vi "GESTORE PROFILI.vi"() -> ()   [LabVIEW 2019]
uses:
  GESTIONE PROFILI Folder/controls/STEP.ctl
  GESTIONE PROFILI Folder/controls/Caratteristiche step.ctl
  TypeDef/PROCEDURE.ctl
  Stato comandi freno.vi
  Stato alimentatore 1.vi
  Global stato profilo.vi
  Acq avvenuta global.vi
  Global CAMBIO CTRL FRENO.vi
  Global Gestione stop se eq termico.vi
  Global procedura abilitata.vi
  Global Fine procedure.vi
  <vilib>/addons/database/NI_Database_API.lvlib
panel:
  in  "To Select Wait":bool=TRUE
  in  "milliseconds to wait":u32=5000
  out "appended array":timestamp[](array[timestamp])
  out "UTILIZZO BANCO":T1(ring)
  out "Settings profilo":T2
  out "Cluster 2":T3
  in  "AGGIORNA SETTINGS AVVIO":bool
  in  "Modalità avvio":T4={"MODALITA' BANCO"=enum."SOLO FRENO", "MODALITA' AVVIO MOTORE"=enum."AVVIO DIRETTO DA LINEA", "MODALITA' AVVIO FRENO"=enum."MARCIA DOPO AVVIO MOTORE", "V avvio[V]"=0.0, "F avvio[Hz]"=0.0, "%V ridotta"=0.0, "C avvio [Nm]"=0.0, "RPM avvio"=0.0, "SERVO AVVIO"=FALSE, "SENSO DI ROTAZIONE"=FALSE}
  in  "NOME PROFILO":string
  in  "CARICA PROFILO":bool
  out "data":T5
  in  "AGGIORNA DATI NOMINALI":bool
  in  "Data":T5
  out "State Called in Queue":string
  in  "EXIT":bool
  in  "Stop Button":bool
  in  "Pause Button":bool
  in  "Play Button":bool
  in  "StatoEsegui":string
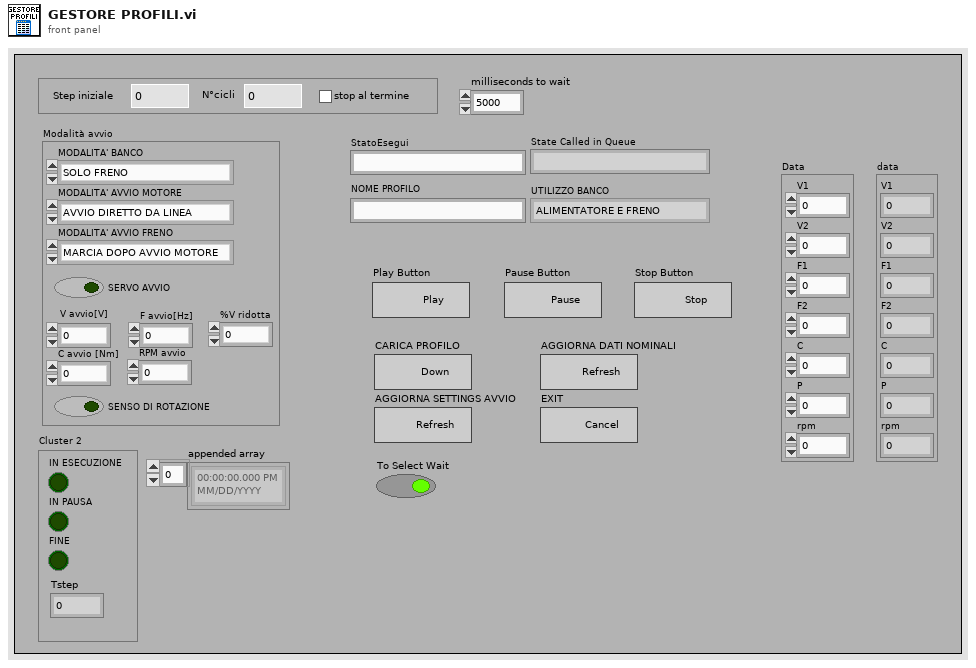
[diagram p1: front panel]
types:
  T1 = enum32{"ALIMENTATORE E FRENO", "SOLO ALIMENTATORE", "SOLO FRENO (TRASCINAMENTO)", "GESTIONE MANUALE", "SOLO ACQUISITORE", "VARIAC"}
  T2 = cluster{"Step iniziale":dbl, "N°cicli":dbl, "stop al termine":bool}
  T3 = cluster{"IN ESECUZIONE":bool, "IN PAUSA":bool, "FINE":bool, "Tstep":dbl}
  T4 = typedef "Modalità avvio.ctl" = cluster{"MODALITA' BANCO":enum32{"ALIMENTATORE E FRENO", "SOLO ALIMENTATORE", "SOLO FRENO", "GESTIONE MANUALE", "SOLO ACQUISITORE", "VARIAC"}, "MODALITA' AVVIO MOTORE":enum32{"AVVIO A TENSIONE RIDOTTA", "AVVIO IN RAMPA", "AVVIO DIRETTO DA ALIM", "AVVIO DIRETTO DA LINEA"}, "MODALITA' AVVIO FRENO":enum32{"MARCIA DOPO AVVIO MOTORE", "MARCIA PRIMA AVVIO"}, "V avvio[V]":dbl, "F avvio[Hz]":dbl, "%V ridotta":dbl, "C avvio [Nm]":dbl, "RPM avvio":dbl, "SERVO AVVIO":bool, "SENSO DI ROTAZIONE":bool}
  T5 = cluster{"V1":dbl, "V2":dbl, "F1":dbl, "F2":dbl, "C":dbl, "P":dbl, "rpm":dbl}
  T6 = cluster{"Message":string, "Message Data":variant}
  T7 = typedef "STEP.ctl" = cluster{"Tipo prova":string, "Misura resistenza ?":bool, "Tempo Step[s]":dbl, "Freno":cluster{"MARCIA":bool, "Control Type":enum32{"Torque [Nm]", "Power [W]", "Speed [RPM]", "Corrente [A]"}, "RIF %":dbl}, "ALIMENTATORE 1":cluster{"MARCIA":bool, "RIF V":dbl, "RIF F":dbl}, "ALIMENTATORE 2":cluster{"MARCIA":bool, "RIF V":dbl, "RIF F":dbl}, "Caratteristiche step":T8}
  T8 = typedef "Caratteristiche step.ctl" = cluster{"Attendi stabilizz.":bool, "Acq. fine step?":bool, "Acq. automatiche":bool, "PID FRENO":bool, "PID ALIMENTATORE 1":bool, "PID ALIMENTATORE 2":bool, "CAMBIA PROVA SE EQ. TERMICO":bool}
  T9 = cluster{"#ripetizione in corso":i32, "Step in corso":i32}
  T10 = cluster{"Array of elements":cluster{"String":string, "variant":variant}[], "Single element":cluster{"String":string, "variant":variant}, "enque at\nopposite end (F)":bool, "no replications (F)":bool}
  T11 = cluster{"N°Acq":i16, "Periodo":dbl, "acq in corso":bool, "Acquisizione":bool, "Slide":u8, "Inserisci Acq.":bool, "Elimina riga":bool, "Acq auto":bool, "Intervallo":dbl}
  T12 = typedef "PROCEDURE.ctl" = enum16{"START", "STOP AUTOMATICO", "STOP FRENO", "ABILITA POTENZA", "DISABILITA POTENZA", "CHIUDI POTENZA", "APRI POTENZA", "MISURA RESISTENZA RESISTOMAT", "PROVA ROTORE BLOCCATO", "MISURA RESISTENZA RES METER", "START AFE ALTERNATORI", "STOP AFE ALTERNATORI", "STOP ALIMENTATORE", "CONFIG CONTROLLO FRENO", "ALLARME", "START PROFILO", "SVUOTA BUFFER PROCEDURE E OPERAZIONI"}
  T13 = cluster{"Step iniziale":i32, "N°cicli":i32, "stop al termine":bool}
  T14 = typedef "Stato inverter selezionato.ctl" = cluster{"Stato comandi freno":T15, "Stato":cluster{"rif C%":dbl, "rif vel%":dbl, "Controllo effettivo":enum32{"Torque [Nm]", "Power [W]", "Speed [RPM]"}, "Controllo desiderato":enum32{"Torque [Nm]", "Power [W]", "Speed [RPM]"}, "Fine rampa C":bool, "Fine rampa RPM":bool, "Senso rotaz":bool, "Start":bool, "C stabile":bool, "P stabile":bool, "RPM stabile":bool}}
  T15 = typedef "Comandi freno.ctl" = cluster{"Control":cluster{"Control Type":enum32{"Torque [Nm]", "Power [W]", "Speed [RPM]", "Corrente [A]"}, "Set":dbl, "Inverti senso di rotazione":bool}, "Start\\stop":cluster{"Start":bool, "STOP":bool}, "Status":cluster{"Ready":bool, "Running":bool, "Regulation":bool}, "PID":bool, "Abilita":cluster{"Abilita":bool}, "Status ref":cluster{"Torque":dbl, "Speed":dbl}}
  T16 = typedef "Comandi_Alimentatore.ctl" = cluster{"RIF 1":dbl, "RIF 2":dbl, "Status":cluster{"Ready":bool, "Running":bool, "Regulation":bool}, "Start\\stop":cluster{"Start":bool, "Stop":bool}, "PID RIF1":bool, "PID RIF2":bool, "Status ref":cluster{"RIF 1":dbl, "RIF 2":dbl}, "Abilita":cluster{"Abilita":bool}}
  T17 = cluster{"RIF 1":dbl, "RIF 2":dbl, "Abilitato":bool, "In marcia":bool, "Fine rampa RIF1":bool, "Fine rampa RIF2":bool, "Vstabile":bool, "F stabile":bool, "PID RIF1":bool, "PID RIF2":bool, "Alimentatore 1":T16}
  T18 = cluster{"RIF 1":dbl, "RIF 2":dbl, "Abilitato":bool, "In marcia":bool, "Fine rampa RIF1":bool, "Fine rampa RIF2":bool, "Vstabile":bool, "F stabile":bool, "PID RIF1":bool, "PID RIF2":bool, "Alimentatore 2":T16}
  T19 = typedef "NI_Database_API.lvlib/Conn ObjectReference.ctl" = refnum<k1>
  T20 = enum32{"Torque [Nm]", "Power [W]", "Speed [RPM]", "Corrente [A]"}
  T21 = cluster{"Caratteristiche step":T8, "Step profilo":string[][]}
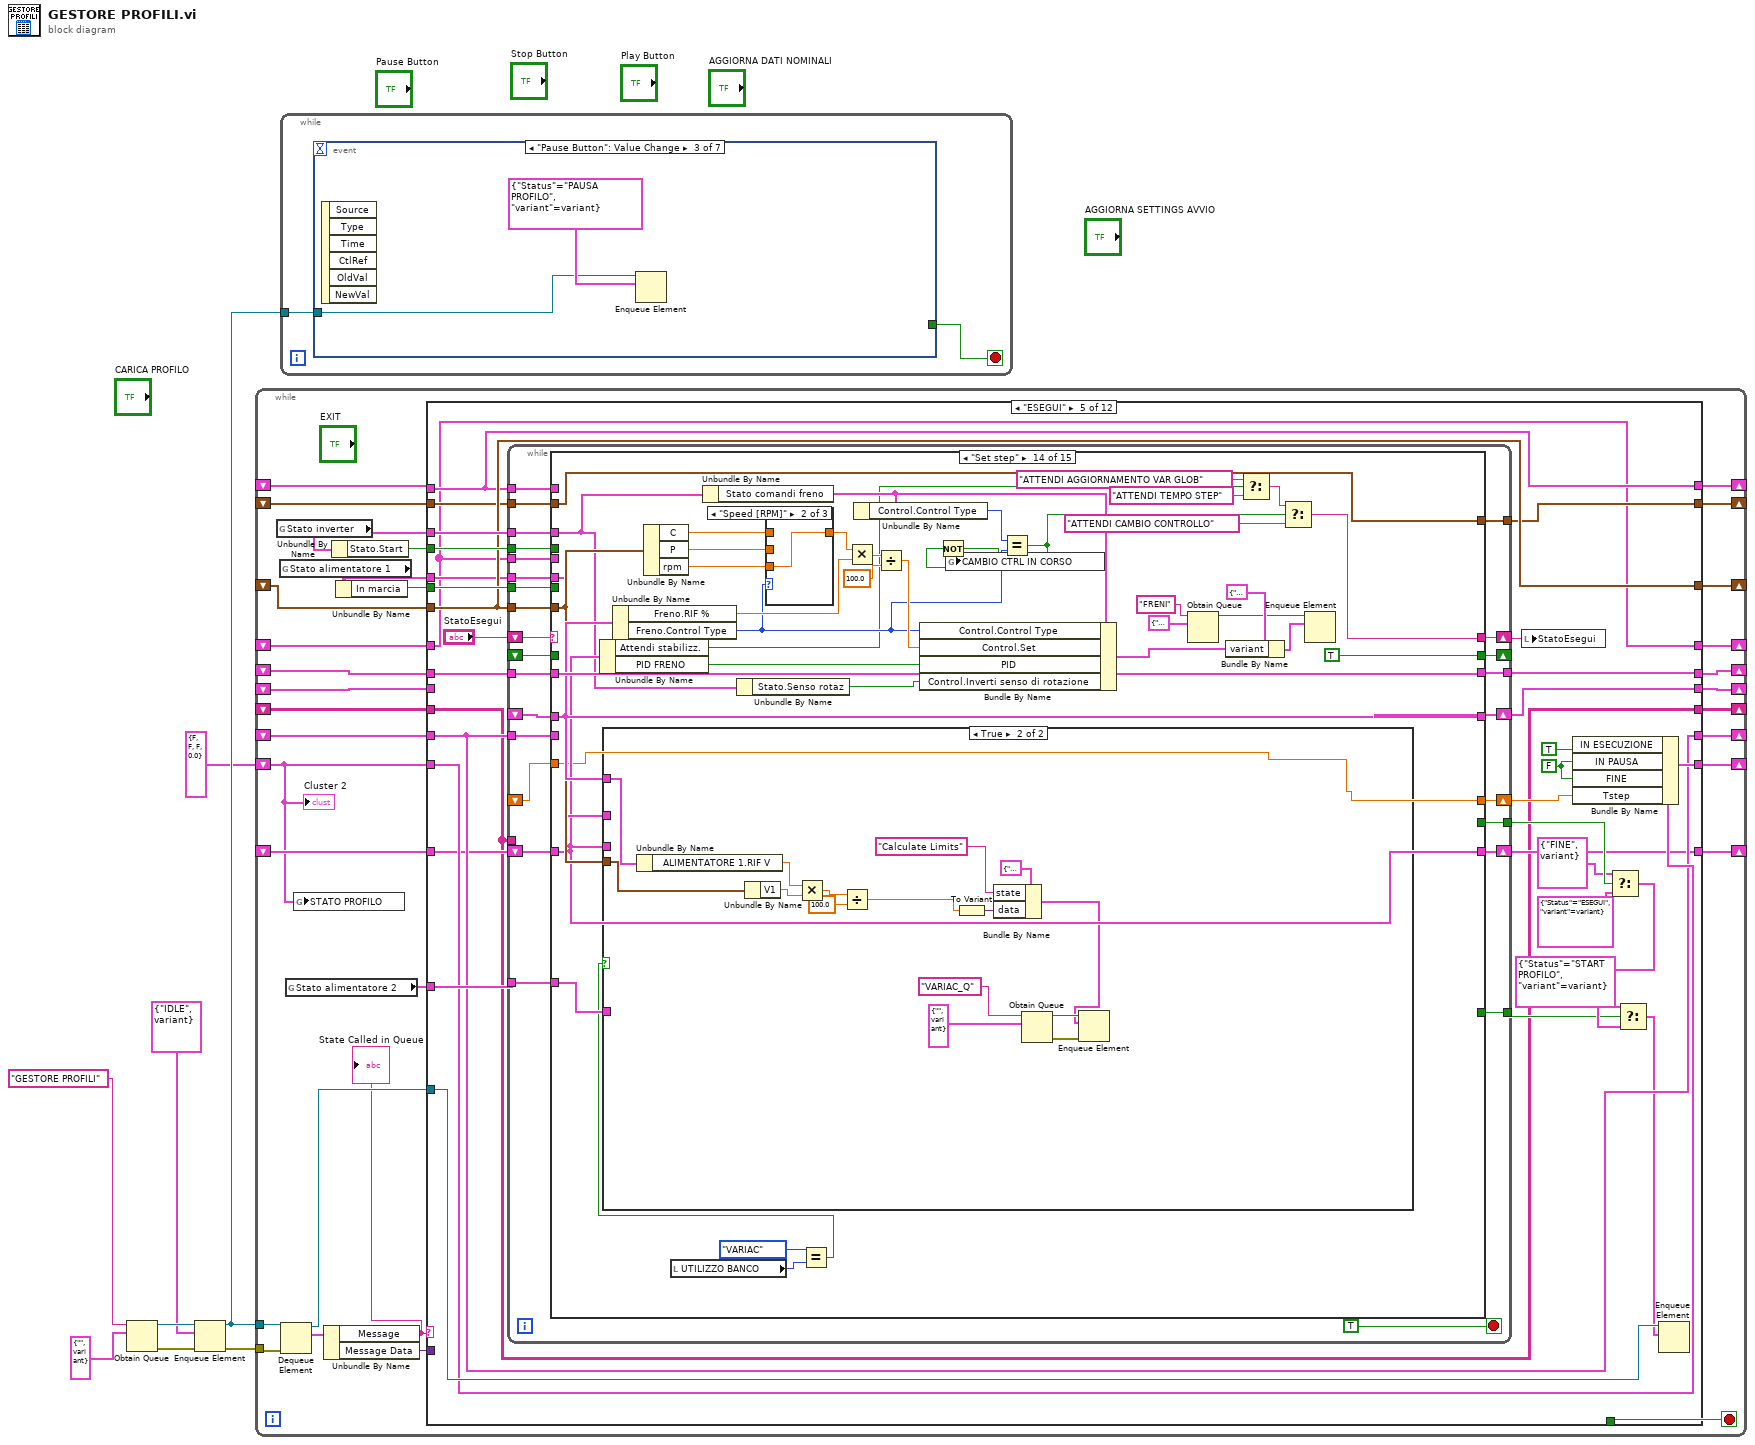
[diagram p0: block diagram]
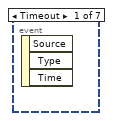
[diagram p2: hidden frame]
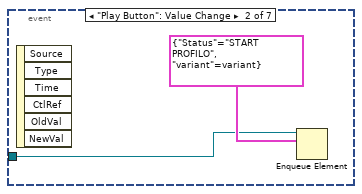
[diagram p3: hidden frame]
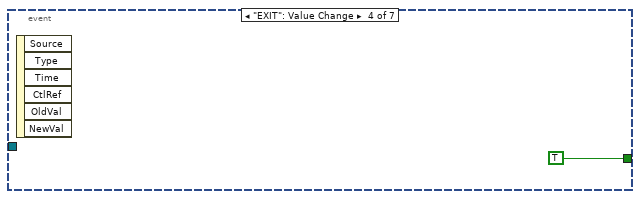
[diagram p4: hidden frame]
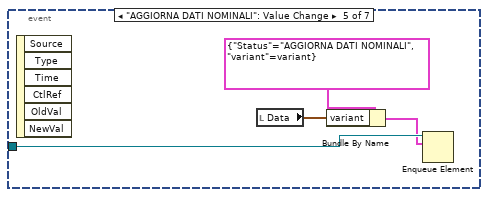
[diagram p5: hidden frame]
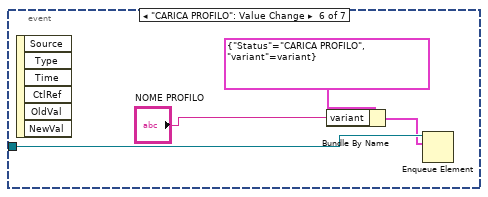
[diagram p6: hidden frame]
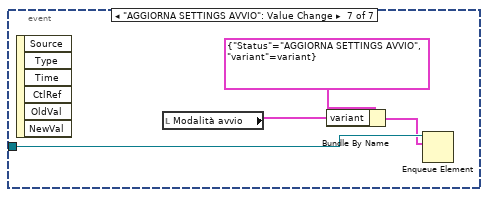
[diagram p7: hidden frame]
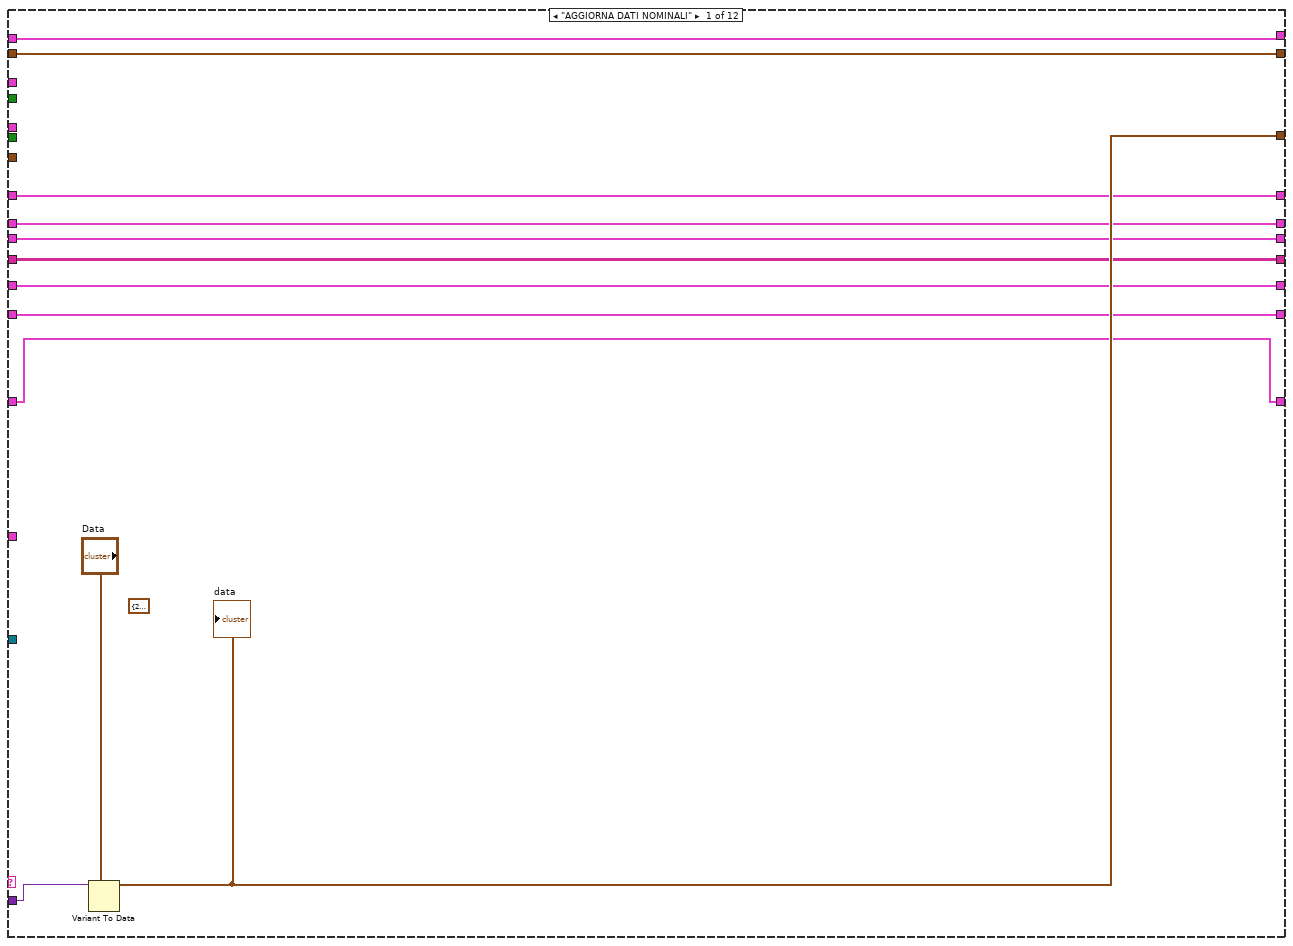
[diagram p8: hidden frame]
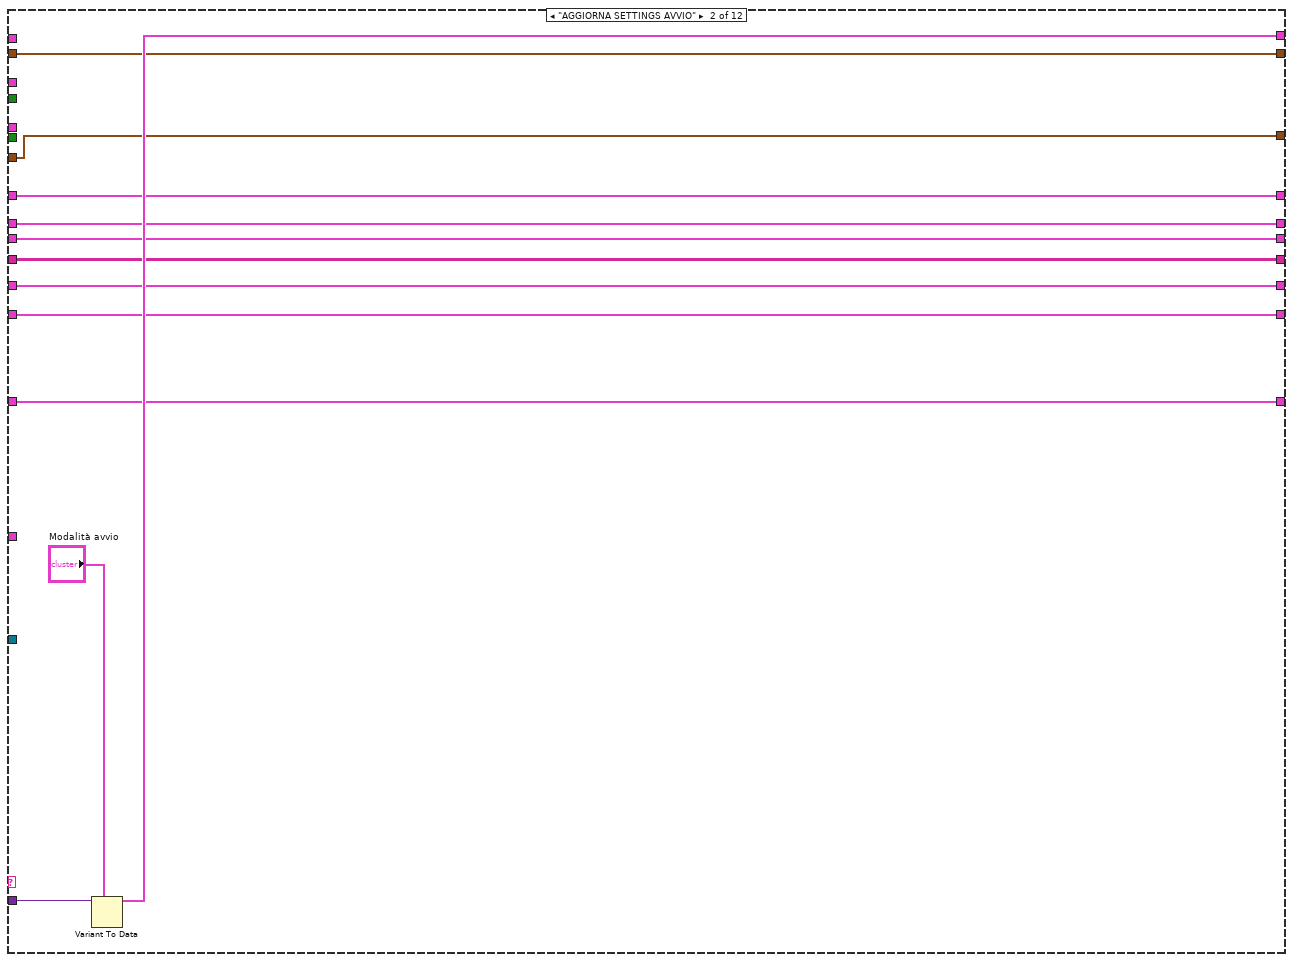
[diagram p9: hidden frame]
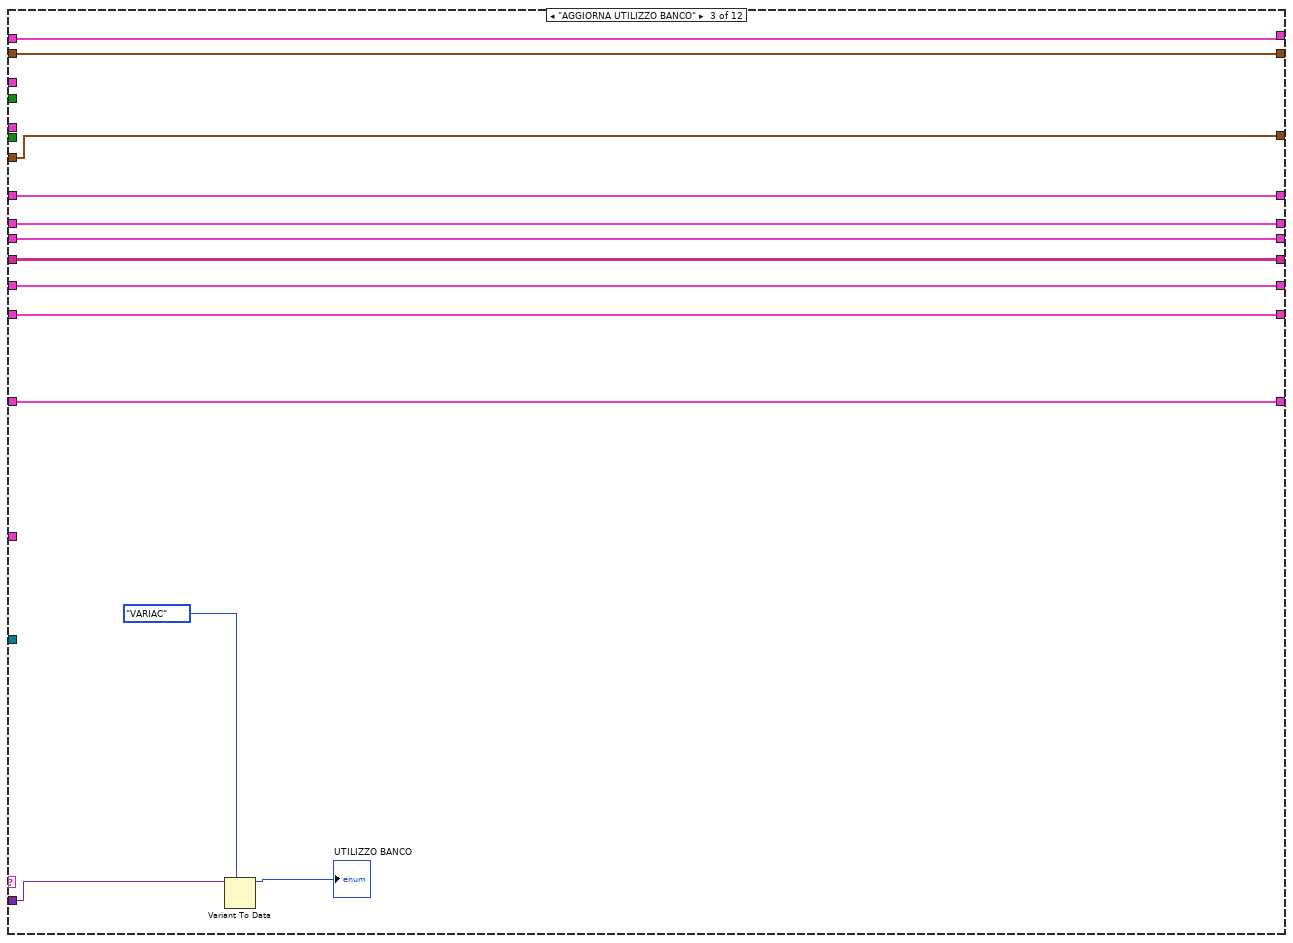
[diagram p10: hidden frame]
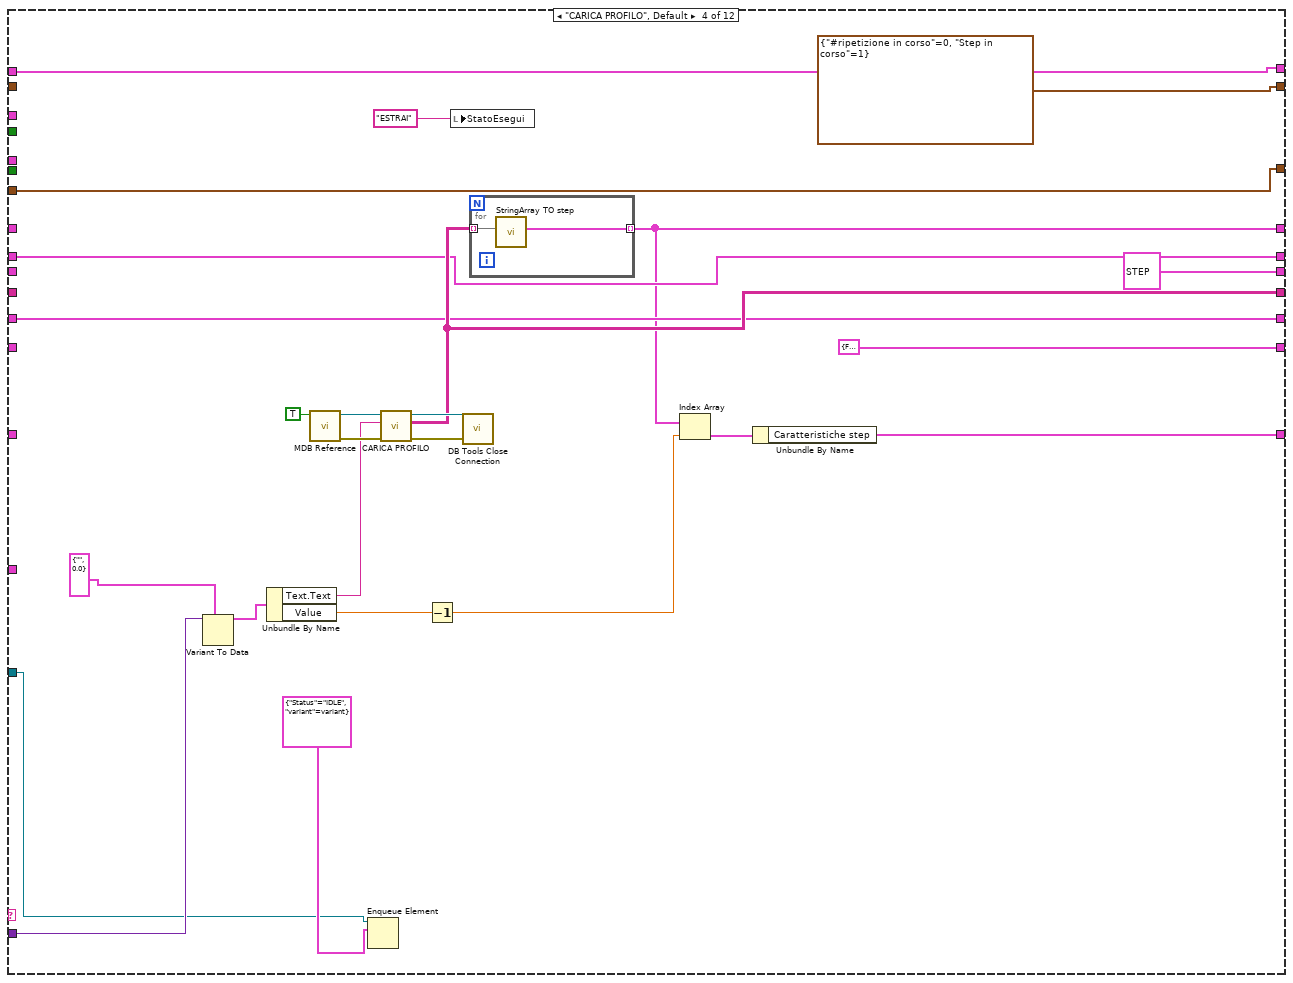
[diagram p11: hidden frame]
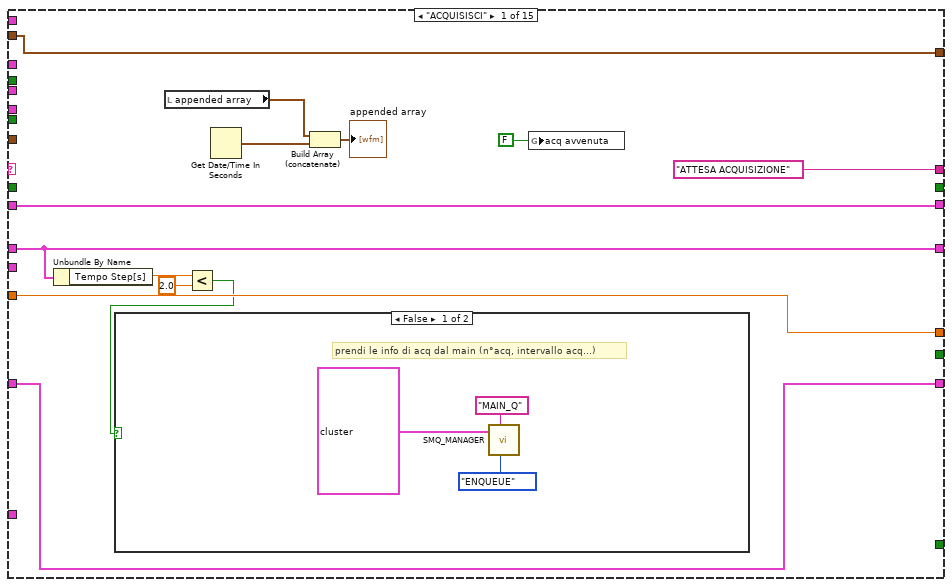
[diagram p12: hidden frame]
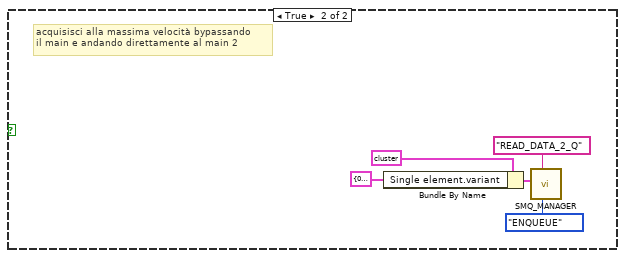
[diagram p13: hidden frame]
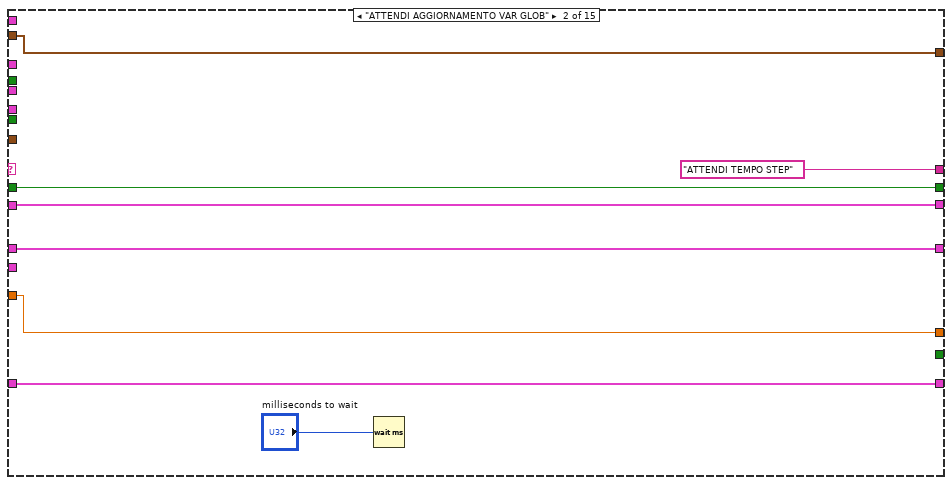
[diagram p14: hidden frame]
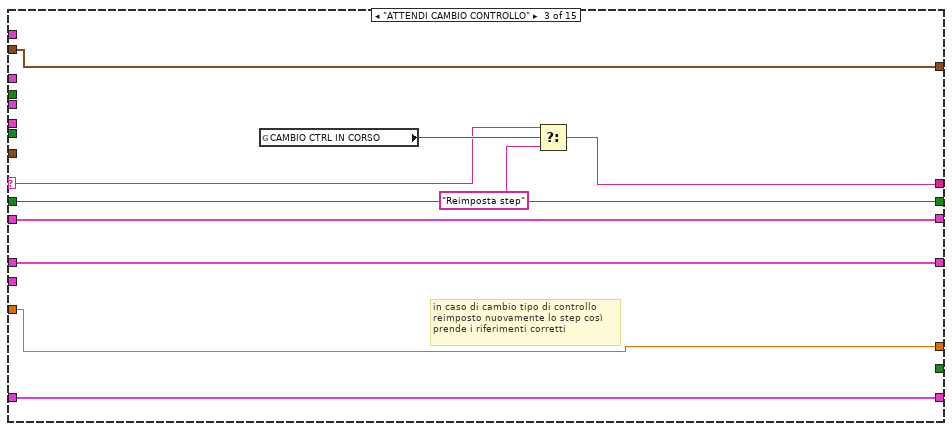
[diagram p15: hidden frame]
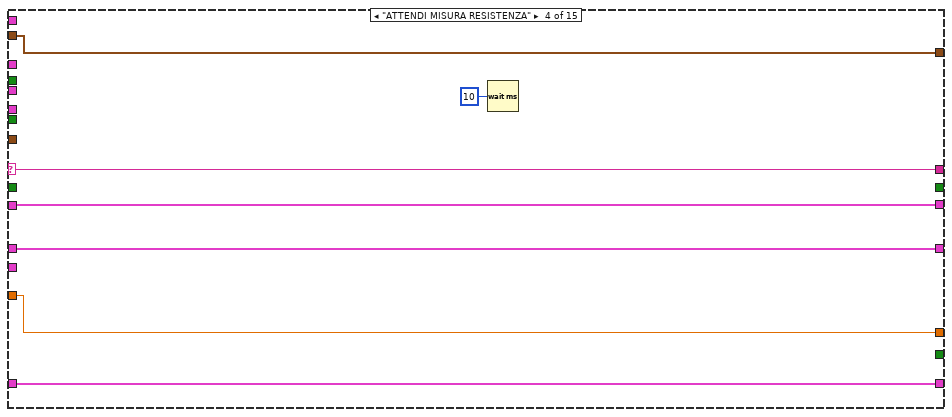
[diagram p16: hidden frame]
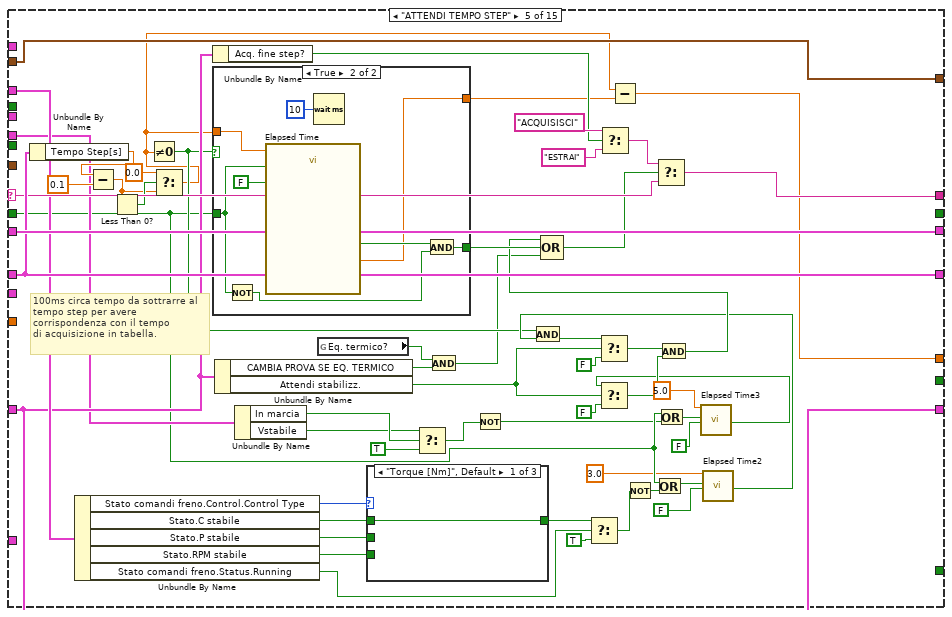
[diagram p17: hidden frame]
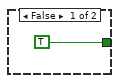
[diagram p20: hidden frame]
diagram:
  n1 = Obtain Queue(name (unnamed)="GESTORE PROFILI", element data type=T6 {"Message"="", "Message Data"=variant} ("Message Cluster")) -> (queue out=w7:refnum<queue>, error out=w8:errorcluster)  [unwired: 3 in, 1 out]
  n2 = Enqueue Element(queue=w7, element=cluster{"Status":string, "variant":variant} {"Status"="IDLE", "variant"=variant}, error in (no error)=w8) -> (queue out=w2:refnum<queue>, error out=w3:errorcluster)  [unwired: 1 in, 1 out]
  n3 = while {
    shift-right: [w40] -> _
    shift-left: _ -> [w39]
    shift-right: [w34] -> _
    shift-left: _ -> [w33]
    tunnel: w2 -> [w32]
    tunnel: w3 -> [w31]
    shift-right: [w25] -> _
    shift-left: _ -> [w24]
    shift-right: [w23] -> _
    shift-left: _ -> [w22]
    shift-right: [w20] -> _
    shift-left: _ -> [w19]
    shift-right: [w18] -> _
    shift-left: _ -> [w17]
    shift-right: [w16] -> _
    shift-left: T3 {"IN ESECUZIONE"=FALSE, "IN PAUSA"=FALSE, "FINE"=FALSE, "Tstep"=0.0} ("STATO PROFILO") -> [w11]
    shift-right: [w15] -> _
    shift-left: _ -> [w14]
    shift-right: [w13] -> _
    shift-left: _ -> [w12]
    shift-right: [w10] -> _
    shift-left: _ -> [w9]
    stop <- w27 stop-if-true
    n4 = global read "Stato comandi freno.vi" "Stato inverter"() -> (w36:T14)
    n5 = global read "Stato alimentatore 1.vi" "Stato alimentatore 1"() -> (w35:T17)
    n6 = Dequeue Element(queue=w32, error in (no error)=w31) -> (queue out=w28:refnum<queue>, element=w30:T6)  [unwired: 1 in, 2 out]
    n7 = global read "Stato alimentatore 1.vi" "Stato alimentatore 2"() -> (w26:T18)
    n8 = global write "Global stato profilo.vi" "STATO PROFILO"(w11) -> ()
    n9 = Unbundle By Name(w30) -> ("Message"=w21:string, "Message Data"=w29:variant)
    "State Called in Queue" <- w21
    n10 = Unbundle By Name(w36) -> ("Stato.Start"=w38:bool)
    n11 = Unbundle By Name(w35) -> ("In marcia"=w37:bool)
    n12 = case shown="\"ESEGUI\"" w21 {
      tunnel: [w45 w61 w69 w90 w135 w594 w611 w625 w646 w651 w672 T7[] []] -> w40
      tunnel: w39 -> [w45 w61 w69 w90 w136 w594 w611 w625 w646 w651 w673 _]
      tunnel: w38 -> [_ _ _ _ w134 _ _ _ _ _ _ _]
      tunnel: w37 -> [_ _ _ _ w133 _ _ _ _ _ _ _]
      tunnel: w36 -> [_ _ _ _ w132 _ _ _ _ _ _ _]
      tunnel: w24 -> [_ w60 w77 w100 w131 w593 w609 w632 w644 w659 w678 w706]
      tunnel: w35 -> [_ _ _ _ w130 _ _ _ _ _ _ _]
      tunnel: w33 -> [w49 _ w70 w102 w129 w595 w612 w633 w647 w653 w671 w699]
      tunnel: [w49 w62 w70 w102 w129 w595 w612 w633 w647 w653 w671 w699] -> w34
      tunnel: w29 -> [w52 w64 w71 w94 _ _ _ _ _ w655 _ _]
      tunnel: w28 -> [_ _ _ w92 w127 _ w610 _ w645 _ w679 w695]
      tunnel: [_ _ _ _ _ w591 _ _ _ _ _ _] -> w27
      tunnel: w26 -> [_ _ _ _ w122 _ _ _ _ _ _ _]
      tunnel: [w50 w60 w77 w100 w131 w593 w609 w632 w644 w659 w678 w706] -> w25
      tunnel: [w48 w59 w76 w85 w106 w592 w599 w626 w643 w658 w670 w705] -> w23
      tunnel: w22 -> [w48 w59 w76 _ w107 w592 w599 w626 w643 w658 w670 w705]
      tunnel: [w47 w58 w75 w91 w105 w590 w608 w624 w642 w657 w677 w704] -> w20
      tunnel: w19 -> [w47 w58 w75 _ w105 w590 w608 w624 w642 w657 w677 w704]
      tunnel: [w46 w57 w74 w87 w114 w589 w605 w623 w641 w656 w665 w703] -> w18
      tunnel: w17 -> [w46 w57 w74 _ w114 w589 w605 w623 w641 w656 w665 w703]
      tunnel: w11 -> [w44 w56 w68 _ w121 w588 w604 w622 w640 w650 w675 w702]
      tunnel: [w44 w56 w68 T3 {"IN ESECUZIONE"=FALSE, "IN PAUSA"=FALSE, "FINE"=FALSE, "Tstep"=0.0} ("STATO PROFILO") w120 w588 w603 w622 w639 w650 w675 w702] -> w16
      tunnel: [w43 w54 w73 w88 w117 w586 w598 w620 w635 w652 w663 w698] -> w15
      tunnel: w14 -> [w43 w54 w73 w88 w117 w586 w598 w620 w635 _ w663 w698]
      tunnel: [w41 w55 w72 T9 {"#ripetizione in corso"=0, "Step in corso"=1} w115 w587 w600 w621 w636 w649 w662 T9 {"#ripetizione in corso"=0, "Step in corso"=1}] -> w13
      tunnel: w12 -> [w41 w55 w72 _ w116 w587 w600 w621 w636 w649 w662 _]
      tunnel: [w42 w53 w67 T7 {"Tipo prova"="[3] ROT. BLOCCATO", "Misura resistenza ?"=FALSE, "Tempo Step[s]"=0.0, "Freno"={"MARCIA"=FALSE, "Control Type"=enum."Torque [Nm]", "RIF %"=0.0}, "ALIMENTATORE 1"={"MARCIA"=FALSE, "RIF V"=0.0, "RIF F"=0.0}, "ALIMENTATORE 2"={"MARCIA"=FALSE, "RIF V"=0.0, "RIF F"=0.0}, "Caratteristiche step"={"Attendi stabilizz."=TRUE, "Acq. fine step?"=TRUE, "Acq. automatiche"=TRUE, "PID FRENO"=TRUE, "PID ALIMENTATORE 1"=TRUE, "PID ALIMENTATORE 2"=FALSE, "CAMBIA PROVA SE EQ. TERMICO"=FALSE}} ("STEP") w108 w585 w596 w619 w634 w648 w666 w694] -> w10
      tunnel: w9 -> [w42 w53 w67 _ _ w585 w596 w619 w634 w648 w666 w694]
      frame "AGGIORNA DATI NOMINALI" {
        (unwired) T5 {"V1"=250.0, "V2"=0.0, "F1"=50.0, "F2"=0.0, "C"=25.0, "P"=10.0, "rpm"=2100.0} ("Cluster")
        n13 = Variant To Data(type="Data", Variant=w52) -> (data=w50:T5)  [unwired: 1 in, 1 out]
        "data" <- w50
      }
      frame "AGGIORNA SETTINGS AVVIO" {
        n14 = Variant To Data(type="Modalità avvio", Variant=w64) -> (data=w62:T4)  [unwired: 1 in, 1 out]
      }
      frame "AGGIORNA UTILIZZO BANCO" {
        n15 = Variant To Data(type=T1."VARIAC" ("MODALITA' UTILIZZO BANCO"), Variant=w71) -> (data=→"UTILIZZO BANCO":T1)  [unwired: 1 in, 1 out]
      }
      frame "CARICA PROFILO", Default {
        n16 = Variant To Data(type=cluster{"Text.Text":string, "Value":dbl} {"Text.Text"="", "Value"=0.0} ("output cluster"), Variant=w94) -> (data=w81:cluster{"Text.Text":string, "Value":dbl})  [unwired: 1 in, 1 out]
        n17 = Unbundle By Name(w81) -> ("Text.Text"=w80:string, "Value"=w79:dbl)
        n18 = call "MDB Reference.vi"("Collaudi T/motori F"=TRUE) -> ("error out"=w98:errorcluster, "Refnum out"=w96:T19)  [unwired: 8 in, 1 out]
        n19 = Enqueue Element(queue=w92, element=cluster{"Status":string, "variant":variant} {"Status"="IDLE", "variant"=variant}) -> ()  [unwired: 2 in, 3 out]
        n20 = call "CARICA PROFILO.vi"("error in (no error)"=w98, "Text.Text"=w80, "Refnum in"=w96) -> ("error out"=w97:errorcluster, "Step profilo"=w91:string[][], "Refnum out"=w95:T19)  [unwired: 3 in, 3 out]
        n21 = Decrement(x=w79) -> (x-1=w78:dbl)
        n22 = local write "StatoEsegui"("ESTRAI" ("StatoEsegui")) -> ()
        n23 = call <vilib>:"DB Tools Close Connection.vi"("error in (no error)"=w97, "connection reference"=w95) -> ()  [unwired: 5 in, 1 out]
        n24 = for {
          tunnel: w91 -> [w104] mode=indexing
          tunnel: [w103] -> w87 mode=indexing
          n25 = call "StringArray TO step.vi"("ItemNames"=w104) -> ("STEP"=w103:T7)  [unwired: 10 in]
        }
        n26 = Index Array(array=w87, index=w78) -> (element=w86:T7)
        n27 = Unbundle By Name(w86) -> ("Caratteristiche step"=w85:T8)
      }
      frame "ESEGUI" {
        w118 = FALSE ("IN PAUSA")
        n28 = while {
          shift-right: [w154] -> w123
          shift-left: "StatoEsegui" -> [w162]
          tunnel: w136 -> [w160]
          tunnel: [w159] -> w135
          shift-right: [w158] -> w108
          shift-left: _ -> [w157]
          tunnel: w134 -> [w156]
          tunnel: w133 -> [w155]
          tunnel: w132 -> [w153]
          tunnel: w131 -> [w152]
          tunnel: w130 -> [w151]
          tunnel: w129 -> [w150]
          tunnel: [w149] -> w128
          shift-right: [w148] -> _
          shift-left: _ -> [w147]
          tunnel: w122 -> [w146]
          tunnel: w117 -> [w144]
          tunnel: w116 -> [w143]
          tunnel: [w142] -> w115
          tunnel: w114 -> [w141]
          tunnel: [w140] -> w111
          shift-right: [w138] -> w106
          shift-left: w107 -> [w145]
          shift-right: [w139] -> w109
          shift-left: _ -> [w137]
          tunnel: w105 -> [_]
          stop <- TRUE stop-if-true
          n29 = case shown="\"Set step\"" w162 {
            selector: w162 -> [_ _ w196 w203 w261 w284 _ w359 w365 _ _ w407 _ _ w583]
            tunnel: w160 -> [w175 w186 w199 w205 w264 w285 w323 w358 w364 w381 w399 w406 w472 w515 w580]
            tunnel: [w175 w186 w199 w205 w264 w285 w331 w358 w364 w381 w399 w406 w472 w515 w580] -> w159
            tunnel: [w166 w185 w200 w206 w263 w286 w290 w357 w363 w375 w398 w405 w439 w505 w579] -> w158
            tunnel: w157 -> [w166 w185 w200 w206 w263 w286 _ w357 w363 w375 w398 w405 w439 w505 w579]
            tunnel: w156 -> [_ _ _ _ _ _ _ _ _ _ _ _ _ _ _]
            tunnel: w155 -> [_ _ _ _ _ _ _ _ _ _ _ _ _ _ _]
            tunnel: ["ATTESA ACQUISIZIONE" ("t") "ATTENDI TEMPO STEP" ("t") w195 w203 w260 w283 w294 w359 w365 w372 "ATTENDI MISURA RESISTENZA" ("t") w407 "ATTENDI AGGIORNAMENTO VAR GLOB" ("t") w489 w582] -> w154
            tunnel: w153 -> [_ _ _ _ w255 _ _ _ _ w379 _ _ w471 w485 _]
            tunnel: w152 -> [_ _ _ _ _ _ _ _ _ w377 _ _ w438 w504 _]
            tunnel: w151 -> [_ _ _ _ w217 _ _ _ _ w378 _ _ w437 w503 _]
            tunnel: w150 -> [_ _ _ _ _ _ _ _ _ w380 _ _ _ _ _]
            tunnel: [_ _ _ _ _ _ _ TRUE _ _ _ _ _ _ _] -> w149
            tunnel: [_ w187 w198 _ _ _ _ _ _ _ _ _ TRUE TRUE _] -> w148
            tunnel: w147 -> [_ w187 w198 _ w216 _ _ _ _ _ _ _ _ _ _]
            tunnel: w146 -> [_ _ _ _ _ _ _ _ _ _ _ _ w436 w502 _]
            tunnel: w145 -> [w171 w189 w193 w207 w253 w278 w311 w354 w361 _ w400 w403 w415 w494 w576]
            tunnel: w144 -> [_ _ _ _ _ _ w336 _ _ _ _ _ _ _ _]
            tunnel: w143 -> [w172 w191 w201 w208 w254 w279 w328 w355 w362 w376 w401 w408 w413 w493 w577]
            tunnel: [w172 w191 w201 w208 w254 w279 w333 w355 w362 w376 w401 w408 w413 w493 w577] -> w142
            tunnel: w141 -> [_ _ _ _ _ _ w332 _ _ _ _ _ _ _ _]
            tunnel: [_ _ _ _ _ _ _ _ _ _ _ TRUE _ _ _] -> w140
            tunnel: [w170 w190 w192 w202 w228 w277 0.0 w353 w360 w371 w393 w402 w409 w483 w575] -> w139
            tunnel: [w171 w189 w193 w207 w253 w278 w311 w354 w361 w374 w400 w403 w415 w494 w576] -> w138
            tunnel: w137 -> [w170 w190 w192 w202 _ w277 _ w353 w360 w371 w393 w402 w409 w483 w575]
            frame "ACQUISISCI" {
              n30 = Unbundle By Name(w166) -> ("Tempo Step[s]"=w165:dbl)
              n31 = local read "appended array"() -> (w167:timestamp[])
              n32 = Less?(x=w165, y=2.0) -> (x < y?=w163:bool)
              n33 = case shown="False" w163 {
                frame False {
                  # "prendi le info di acq dal main (n°acq, intervallo acq...)"
                  n34 = call <userlib>:"SMQ_MANAGER.vi"("Function"=enum16{"INITIALIZE", "ENQUEUE", "STOP ALL"}."ENQUEUE", "Queue name"="MAIN_Q", "Enqueue cluster"=T10 {"Array of elements"=[], "Single element"={"String"="ACQUISISCI", "variant"=variant}, "enque at\nopposite end (F)"=FALSE, "no replications (F)"=FALSE}) -> ()  [unwired: 8 in, 1 out]
                }
                frame True {
                  # "acquisisci alla massima velocità bypassando\nil main e andando direttamente al main 2"
                  n35 = Bundle By Name(cluster=T10 {"Array of elements"=[], "Single element"={"String"="START ACQ", "variant"=variant}, "enque at\nopposite end (F)"=FALSE, "no replications (F)"=FALSE} ("Enqueue cluster"), "Single element.variant"=T11 {"N°Acq"=0, "Periodo"=0.0, "acq in corso"=FALSE, "Acquisizione"=FALSE, "Slide"=2, "Inserisci Acq."=FALSE, "Elimina riga"=FALSE, "Acq auto"=FALSE, "Intervallo"=5.0} ("Acquisizioni")) -> (w180:T10)
                  n36 = call <userlib>:"SMQ_MANAGER.vi"("Function"=enum16{"INITIALIZE", "ENQUEUE", "STOP ALL"}."ENQUEUE", "Queue name"="READ_DATA_2_Q", "Enqueue cluster"=w180) -> ()  [unwired: 8 in, 1 out]
                }
              }
              n37 = Get Date/Time In Seconds() -> (seconds since 1Jan1904=w169:timestamp)
              n38 = Build Array (concatenate)(w167, w169) -> (→"appended array":timestamp[])
              n39 = global write "Acq avvenuta global.vi" "acq avvenuta"(FALSE) -> ()
            }
            frame "ATTENDI AGGIORNAMENTO VAR GLOB" {
              n40 = Wait (ms)(milliseconds to wait="milliseconds to wait") -> ()  [unwired: 1 out]
            }
            frame "ATTENDI CAMBIO CONTROLLO" {
              # "in caso di cambio tipo di controllo\nreimposto nuovamente lo step così\nprende i riferimenti corretti"
              n41 = global read "Global CAMBIO CTRL FRENO.vi" "CAMBIO CTRL IN CORSO"() -> (w197:bool)
              n42 = Select(t=w196, s=w197, f="Reimposta step") -> (s? t:f=w195:string)
            }
            frame "ATTENDI MISURA RESISTENZA" {
              n43 = Wait (ms)(milliseconds to wait=u32 10) -> ()  [unwired: 1 out]
            }
            frame "ATTENDI TEMPO STEP" {
              # "100ms circa tempo da sottrarre al\ntempo step per avere\ncorrispondenza con il tempo\ndi acquisizione in tabella."
              n44 = Unbundle By Name(w263) -> ("Tempo Step[s]"=w226:dbl)
              n45 = Unbundle By Name(w255) -> ("Stato comandi freno.Control.Control Type"=w252:T20, "Stato.C stabile"=w251:bool, "Stato.P stabile"=w250:bool, "Stato.RPM stabile"=w249:bool, "Stato comandi freno.Status.Running"=w242:bool)
              n46 = Subtract(x=w226, y=0.1) -> (x-y=w223:dbl)
              n47 = Less Than 0?(x=w223) -> (x < 0?=w224:bool)
              n48 = Select(t=0.0, s=w224, f=w223) -> (s? t:f=w221:dbl)
              n49 = Not Equal To 0?(x=w221) -> (x != 0?=w227:bool)
              n50 = Unbundle By Name(w253) -> ("Acq. fine step?"=w256:bool)
              n51 = case shown="True" w227 {
                tunnel: w221 -> [_ w276]
                tunnel: [TRUE ("Time has Elapsed") w272] -> w262
                tunnel: w216 -> [_ w271]
                tunnel: [_ w269] -> w229
                frame False {
                }
                frame True {
                  n52 = Not(x=w271) -> (.not. x?=w270:bool)
                  n53 = call "Elapsed Time"("Time Target (s)"=w276, "Reset"=w271, "Auto Reset"=FALSE) -> ("Elapsed Time (s)"=w269:dbl, "Time has Elapsed"=w275:bool)  [unwired: 9 in, 6 out]
                  n54 = Wait (ms)(milliseconds to wait=u32 10) -> ()  [unwired: 1 out]
                  n55 = And(x=w275, y=w270) -> (x .and. y?=w272:bool)
                }
              }
              n56 = Unbundle By Name(w253) -> ("CAMBIA PROVA SE EQ. TERMICO"=w220:bool, "Attendi stabilizz."=w237:bool)
              n57 = Unbundle By Name(w217) -> ("In marcia"=w239:bool, "Vstabile"=w238:bool)
              n58 = global read "Global Gestione stop se eq termico.vi" "Eq. termico?"() -> (w219:bool)
              n59 = case shown="\"Torque [Nm]\", Default" w252 {
                tunnel: w251 -> [w265 _ _]
                tunnel: w250 -> [_ w266 _]
                tunnel: w249 -> [_ _ w267]
                tunnel: [w265 w266 w267] -> w243
                frame "Torque [Nm]", Default {
                }
                frame "Power [W]" {
                }
                frame "Speed [RPM]" {
                }
              }
              n60 = Select(t=w238, s=w239, f=TRUE) -> (s? t:f=w212:bool)
              n61 = And(x=w219, y=w220) -> (x .and. y?=w218:bool)
              n62 = Not(x=w212) -> (.not. x?=w211:bool)
              n63 = Select(t=w243, s=w242, f=TRUE) -> (s? t:f=w232:bool)
              n64 = Select(t="ACQUISISCI", s=w256, f="ESTRAI" ("t")) -> (s? t:f=w258:string)
              n65 = Subtract(x=w221, y=w229) -> (x-y=w228:dbl)
              n66 = Not(x=w232) -> (.not. x?=w235:bool)
              n67 = Or(x=w216, y=w235) -> (x .or. y?=w233:bool)
              n68 = Or(x=w216, y=w211) -> (x .or. y?=w215:bool)
              n69 = call "Elapsed Time3"("Time Target (s)"=5.0, "Reset"=w215, "Auto Reset"=FALSE) -> ("Time has Elapsed"=w210:bool)  [unwired: 9 in, 7 out]
              n70 = Select(t=w210, s=w237, f=FALSE) -> (s? t:f=w245:bool)
              n71 = call "Elapsed Time2"("Time Target (s)"=3.0, "Reset"=w233, "Auto Reset"=FALSE) -> ("Time has Elapsed"=w231:bool)  [unwired: 9 in, 7 out]
              n72 = And(x=w227, y=w231) -> (x .and. y?=w230:bool)
              n73 = Select(t=w230, s=w237, f=FALSE) -> (s? t:f=w244:bool)
              n74 = And(x=w244, y=w245) -> (x .and. y?=w236:bool)
              n75 = Compound Arithmetic op=OR(w236, w262, w218) -> (w248:bool)
              n76 = Select(t=w258, s=w248, f=w261) -> (s? t:f=w260:string)
            }
            frame "ATTESA ACQUISIZIONE" {
              n77 = global read "Acq avvenuta global.vi" "acq avvenuta"() -> (w280:bool)
              n78 = Wait (ms)(milliseconds to wait=u32 10) -> ()  [unwired: 1 out]
              n79 = Select(t="ESTRAI", s=w280, f=w284) -> (s? t:f=w283:string)
            }
            frame "ESTRAI" {
              w310 = 1 ("length (rest)")
              # "extract"
              n80 = Unbundle By Name(w336) -> ("Step iniziale"=w320:i32, "N°cicli"=w327:i32)
              n81 = Unbundle By Name(w328) -> ("#ripetizione in corso"=w313:i32)
              n82 = Decrement(x=w320) -> (x-1=w315:i32)
              n83 = Decrement(x=w327) -> (x-1=w314:i32)
              n84 = Equal To 0?(x=w313) -> (x = 0?=w322:bool)
              n85 = Select(t=w315, s=w322, f=0) -> (s? t:f=w316:i32)
              n86 = Delete From Array(array=w323, length=1, index=w316) -> (deleted portion=w341:T7[], array with subset deleted=w331:T7[])
              n87 = Array Size(array=w331) -> (size(s)=w319:i32)
              n88 = Array Size(array=w332) -> (size(s)=w330:i32)
              n89 = Index Array(array=w341) -> (element=w290:T7)  [unwired: 1 in]
              n90 = Unbundle By Name(w290) -> ("Caratteristiche step"=w289:T8)
              n91 = Empty Array?(array=w341) -> (empty?=w335:bool)
              n92 = Subtract(x=w330, y=w319) -> (x-y=w317:i32)
              n93 = Unbundle By Name(w290) -> ("Caratteristiche step.CAMBIA PROVA SE EQ. TERMICO"=w297:bool)
              n94 = global read "Global procedura abilitata.vi" "Prova selezionata"() -> (w308:i8)
              n95 = Increment(x=w313) -> (x+1=w312:i32)
              n96 = Unbundle By Name(w290) -> ("Tipo prova"=w309:string)
              n97 = Greater Or Equal?(x=w313, y=w314) -> (x >= y?=w302:bool)
              n98 = case shown="False" w335 {
                tunnel: w328 -> [w348 w352]
                tunnel: [w348 w349] -> w334
                frame False {
                }
                frame True {
                  n99 = Unbundle By Name(w352) -> ("#ripetizione in corso"=w351:i32)
                  n100 = Increment(x=w351) -> (x+1=w350:i32)
                  n101 = Bundle By Name(cluster=w352, "#ripetizione in corso"=w350) -> (w349:T9)
                }
              }
              n102 = Add(x=w317, y=w316) -> (x+y=w318:i32)
              n103 = Decrement(x=w318) -> (x-1=w324:i32)
              n104 = Build Array(w324, w312) -> (w288:i32[])
              n105 = String Subset(string=w309, offset (0)=w310, length (rest)=w310) -> (substring=w301:string)
              n106 = Bundle(w288, "Caratteristiche step"=w289) -> (w287:cluster{i32[], "Caratteristiche step":T8})  [unwired: 1 in]
              n107 = Not Equal?(x="-", y=w301) -> (x != y?=w303:bool)
              n108 = Empty String/Path?(string/path=w301) -> (empty?=w300:bool)
              n109 = Decimal String To Number(string=w301) -> (number=w306:i32)  [unwired: 2 in, 1 out]
              n110 = Not Equal?(x=w306, y=w308) -> (x != y?=w307:bool)
              n111 = Not(x=w300) -> (.not. x?=w299:bool)
              n112 = global read "Global Gestione stop se eq termico.vi" "Eq. termico?"() -> (w296:bool)
              n113 = Bundle By Name(cluster=T10 {"Array of elements"=[], "Single element"={"String"="AGGIORNA N STEP PROFILO", "variant"=variant}, "enque at\nopposite end (F)"=FALSE, "no replications (F)"=FALSE} ("Enqueue cluster"), "Single element.variant"=w287) -> (w337:T10)
              n114 = Compound Arithmetic op=AND(w299, w307, w303) -> (w304:bool)
              n115 = case shown="True" w304 {
                tunnel: w306 -> [_ w343]
                frame False {
                }
                frame True {
                  # "scelta prova"
                  n116 = Bundle By Name(cluster=T10 {"Array of elements"=[], "Single element"={"String"="SCELTA PROVA", "variant"=variant}, "enque at\nopposite end (F)"=FALSE, "no replications (F)"=FALSE} ("Enqueue cluster"), "Single element.variant"=w343) -> (w344:T10)
                  n117 = call <userlib>:"SMQ_MANAGER.vi"("Function"=enum16{"INITIALIZE", "ENQUEUE", "STOP ALL"}."ENQUEUE", "Queue name"="MAIN2_Q", "Enqueue cluster"=w344) -> ()  [unwired: 8 in, 1 out]
                }
              }
              n118 = Select(t="FINE", s=w302, f="RIPETI PROFILO") -> (s? t:f=w329:string)
              n119 = And(x=w296, y=w297) -> (x .and. y?=w292:bool)
              n120 = Bundle By Name(cluster=w334, "Step in corso"=w318) -> (w333:T9)
              n121 = call <userlib>:"SMQ_MANAGER.vi"("Function"=enum16{"INITIALIZE", "ENQUEUE", "STOP ALL"}."ENQUEUE", "Queue name"="MAIN2_Q", "Enqueue cluster"=w337) -> ()  [unwired: 8 in, 1 out]
              n122 = Select(t="ESTRAI", s=w292, f="IMPOSTA") -> (s? t:f=w291:string)
              n123 = Select(t=w329, s=w335, f=w291) -> (s? t:f=w294:string)
            }
            frame "FINE" {
            }
            frame "False", Default {
            }
            frame "IMPOSTA" {
              # "#TODO NEED TO CONFIGURE FOR VARIAC"
              n124 = Unbundle By Name(w375) -> ("Misura resistenza ?"=w373:bool, "Caratteristiche step"=w374:T8, "Caratteristiche step.Acq. automatiche"=w366:bool)
              n125 = case shown="False" w373 {
                tunnel: w380 -> [w388 _]
                tunnel: w379 -> [w387 _]
                tunnel: w378 -> [w386 _]
                tunnel: w377 -> [w385 _]
                tunnel: w375 -> [w384 _]
                tunnel: [w383 "MISURA RESISTENZA" ("t")] -> w372
                frame False {
                  n126 = local read "UTILIZZO BANCO"() -> (w382:T1)
                  n127 = call "Valuta procedure start stop.vi"("UTILIZZO BANCO"=w382, "Modalità avvio"=w388, "Stato alimentatore 1"=w386, "Stato inverter"=w387, "NUOVO STEP"=w384, "Cluster"=w385) -> ("Prosegui"=w391:bool)  [unwired: 5 in]
                  n128 = Select(t="Set step", s=w391, f="Wait procedura") -> (s? t:f=w383:string)
                }
                frame True {
                }
              }
              n129 = Bundle By Name(cluster=T10 {"Array of elements"=[], "Single element"={"String"="AGGIORNA ACQ AUTO", "variant"=variant}, "enque at\nopposite end (F)"=FALSE, "no replications (F)"=FALSE} ("Enqueue cluster"), "Single element.variant"=w366) -> (w367:T10)
              n130 = call <userlib>:"SMQ_MANAGER.vi"("Function"=enum16{"INITIALIZE", "ENQUEUE", "STOP ALL"}."ENQUEUE", "Queue name"="MAIN_Q", "Enqueue cluster"=w367) -> ()  [unwired: 8 in, 1 out]
            }
            frame "MISURA RESISTENZA" {
              n131 = call <userlib>:"SMQ_MANAGER.vi"("Function"=enum16{"INITIALIZE", "ENQUEUE", "STOP ALL"}."ENQUEUE", "Queue name"="MAIN_Q", "Enqueue cluster"=T10 {"Array of elements"=[], "Single element"={"String"="MISURA RESISTENZA RESISTOMAT", "variant"=variant}, "enque at\nopposite end (F)"=FALSE, "no replications (F)"=FALSE}) -> ()  [unwired: 8 in, 1 out]
            }
            frame "RIPETI PROFILO" {
            }
            frame "Reimposta step" {
              (unwired) "ATTENDI TEMPO STEP" ("t")
              w450 = 100.0 ("y")
              w452 = 100.0 ("y")
              n132 = Unbundle By Name(w439) -> ("ALIMENTATORE 1.MARCIA"=w455:bool, "ALIMENTATORE 1.RIF V"=w454:dbl, "ALIMENTATORE 1.RIF F"=w453:dbl)
              n133 = Unbundle By Name(w437) -> ("Alimentatore 1"=w462:T16)
              n134 = Unbundle By Name(w439) -> ("ALIMENTATORE 2.MARCIA"=w447:bool, "ALIMENTATORE 2.RIF V"=w448:dbl, "ALIMENTATORE 2.RIF F"=w449:dbl)
              n135 = Unbundle By Name(w436) -> ("Alimentatore 2"=w440:T16)
              n136 = Unbundle By Name(w415) -> ("PID ALIMENTATORE 1"=w414:bool)
              n137 = Unbundle By Name(w415) -> ("PID ALIMENTATORE 1"=w416:bool)
              n138 = Unbundle By Name(w439) -> ("Freno.RIF %"=w467:dbl, "Freno.Control Type"=w411:T20)
              n139 = Unbundle By Name(w415) -> ("PID FRENO"=w417:bool)
              n140 = Unbundle By Name(w438) -> ("C"=w470:dbl, "P"=w469:dbl, "rpm"=w468:dbl)
              n141 = Unbundle By Name(w471) -> ("Stato comandi freno"=w412:T15)
              n142 = Unbundle By Name(w438) -> ("V1"=w461:dbl, "F1"=w460:dbl)
              n143 = Unbundle By Name(w438) -> ("V2"=w441:dbl, "F2"=w442:dbl)
              n144 = case shown="\"Speed [RPM]\"" w411 {
                tunnel: w470 -> [w473 _ _]
                tunnel: w469 -> [_ _ w475]
                tunnel: w468 -> [_ w474 _]
                tunnel: [w473 w474 w475] -> w466
                frame "Torque [Nm]", Default {
                }
                frame "Speed [RPM]" {
                }
                frame "Power [W]" {
                }
              }
              n145 = Multiply(x=w454, y=w461) -> (x*y=w459:dbl)
              n146 = Multiply(x=w453, y=w460) -> (x*y=w457:dbl)
              n147 = Multiply(x=w448, y=w441) -> (x*y=w443:dbl)
              n148 = Multiply(x=w449, y=w442) -> (x*y=w445:dbl)
              n149 = Multiply(x=w466, y=w467) -> (x*y=w465:dbl)
              n150 = Divide(x=w465, y=100.0) -> (x/y=w463:dbl)
              n151 = Divide(x=w459, y=w452) -> (x/y=w458:dbl)
              n152 = Divide(x=w457, y=w452) -> (x/y=w456:dbl)
              n153 = Divide(x=w443, y=w450) -> (x/y=w444:dbl)
              n154 = Divide(x=w445, y=w450) -> (x/y=w446:dbl)
              n155 = Bundle By Name(cluster=w412, "Control.Control Type"=w411, "Control.Set"=w463, "PID"=w417) -> (w430:T15)
              n156 = Bundle By Name(cluster=w462, "Start\\stop.Start"=w455, "RIF 1"=w458, "RIF 2"=w456, "PID RIF1"=w416, "PID RIF2"=w416) -> (w424:T16)
              n157 = Bundle By Name(cluster=w440, "Start\\stop.Start"=w447, "RIF 1"=w444, "RIF 2"=w446, "PID RIF1"=w414, "PID RIF2"=w414) -> (w418:T16)
              n158 = Obtain Queue(name (unnamed)="FRENI", element data type=T6 {"Message"="", "Message Data"=variant} ("Message Cluster")) -> (queue out=w434:refnum<queue>)  [unwired: 3 in, 2 out]
              n159 = Obtain Queue(name (unnamed)="ALIMENTATORE 1", element data type=T6 {"Message"="", "Message Data"=variant} ("Message Cluster")) -> (queue out=w428:refnum<queue>)  [unwired: 3 in, 2 out]
              n160 = Obtain Queue(name (unnamed)="ALIMENTATORE 2", element data type=T6 {"Message"="", "Message Data"=variant} ("Message Cluster")) -> (queue out=w420:refnum<queue>)  [unwired: 3 in, 2 out]
              n161 = Bundle By Name(cluster=cluster{"Status":string, "variant":variant} {"Status"="AGGIORNA COMANDI FRENO", "variant"=variant}, "variant"=w430) -> (w431:cluster{"Status":string, "variant":variant})
              n162 = Bundle By Name(cluster=cluster{"Status":string, "variant":variant} {"Status"="AGGIORNA COMANDI ALIMENTATORE", "variant"=variant}, "variant"=w424) -> (w425:cluster{"Status":string, "variant":variant})
              n163 = Bundle By Name(cluster=cluster{"Status":string, "variant":variant} {"Status"="AGGIORNA COMANDI ALIMENTATORE", "variant"=variant}, "variant"=w418) -> (w423:cluster{"Status":string, "variant":variant})
              n164 = Enqueue Element(queue=w434, element=w431) -> ()  [unwired: 2 in, 3 out]
              n165 = Enqueue Element(queue=w428, element=w425) -> ()  [unwired: 2 in, 3 out]
              n166 = Enqueue Element(queue=w420, element=w423) -> ()  [unwired: 2 in, 3 out]
            }
            frame "Set step" {
              n167 = Unbundle By Name(w494) -> ("Attendi stabilizz."=w479:bool, "PID FRENO"=w495:bool)
              n168 = Unbundle By Name(w505) -> ("Freno.RIF %"=w511:dbl, "Freno.Control Type"=w490:T20)
              n169 = Unbundle By Name(w504) -> ("C"=w514:dbl, "P"=w513:dbl, "rpm"=w512:dbl)
              n170 = local read "UTILIZZO BANCO"() -> (w477:T1)
              n171 = Unbundle By Name(w485) -> ("Stato comandi freno"=w492:T15)
              n172 = Unbundle By Name(w485) -> ("Stato.Senso rotaz"=w484:bool)
              n173 = case shown="\"Speed [RPM]\"" w490 {
                tunnel: w514 -> [w572 _ _]
                tunnel: w513 -> [_ _ w574]
                tunnel: w512 -> [_ w573 _]
                tunnel: [w572 w573 w574] -> w510
                frame "Torque [Nm]", Default {
                }
                frame "Speed [RPM]" {
                }
                frame "Power [W]" {
                }
              }
              n174 = Equal?(x=T1."VARIAC" ("UTILIZZO BANCO"), y=w477) -> (x = y?=w476:bool)
              n175 = case shown="True" w476 {
                tunnel: w505 -> [w534 w563]
                tunnel: w504 -> [w533 w562]
                tunnel: w503 -> [w532 _]
                tunnel: w502 -> [w531 _]
                tunnel: w494 -> [w517 _]
                frame False {
                  w545 = 100.0 ("y")
                  w546 = 100.0 ("y")
                  n176 = Unbundle By Name(w534) -> ("ALIMENTATORE 1.MARCIA"=w549:bool, "ALIMENTATORE 1.RIF V"=w548:dbl, "ALIMENTATORE 1.RIF F"=w547:dbl)
                  n177 = Unbundle By Name(w532) -> ("Alimentatore 1"=w556:T16)
                  n178 = Unbundle By Name(w534) -> ("ALIMENTATORE 2.MARCIA"=w542:bool, "ALIMENTATORE 2.RIF V"=w543:dbl, "ALIMENTATORE 2.RIF F"=w544:dbl)
                  n179 = Unbundle By Name(w531) -> ("Alimentatore 2"=w535:T16)
                  n180 = Unbundle By Name(w517) -> ("PID ALIMENTATORE 1"=w516:bool)
                  n181 = Unbundle By Name(w517) -> ("PID ALIMENTATORE 1"=w518:bool)
                  n182 = Unbundle By Name(w533) -> ("V1"=w555:dbl, "F1"=w554:dbl)
                  n183 = Unbundle By Name(w533) -> ("V2"=w536:dbl, "F2"=w537:dbl)
                  n184 = Multiply(x=w548, y=w555) -> (x*y=w553:dbl)
                  n185 = Multiply(x=w547, y=w554) -> (x*y=w551:dbl)
                  n186 = Multiply(x=w543, y=w536) -> (x*y=w538:dbl)
                  n187 = Multiply(x=w544, y=w537) -> (x*y=w540:dbl)
                  n188 = Divide(x=w553, y=w546) -> (x/y=w552:dbl)
                  n189 = Divide(x=w551, y=w546) -> (x/y=w550:dbl)
                  n190 = Divide(x=w538, y=w545) -> (x/y=w539:dbl)
                  n191 = Divide(x=w540, y=w545) -> (x/y=w541:dbl)
                  n192 = Bundle By Name(cluster=w556, "Start\\stop.Start"=w549, "RIF 1"=w552, "RIF 2"=w550, "PID RIF1"=w518, "PID RIF2"=w518) -> (w525:T16)
                  n193 = Bundle By Name(cluster=w535, "Start\\stop.Start"=w542, "RIF 1"=w539, "RIF 2"=w541, "PID RIF1"=w516, "PID RIF2"=w516) -> (w519:T16)
                  n194 = Obtain Queue(name (unnamed)="ALIMENTATORE 1", element data type=T6 {"Message"="", "Message Data"=variant} ("Message Cluster")) -> (queue out=w529:refnum<queue>)  [unwired: 3 in, 2 out]
                  n195 = Obtain Queue(name (unnamed)="ALIMENTATORE 2", element data type=T6 {"Message"="", "Message Data"=variant} ("Message Cluster")) -> (queue out=w521:refnum<queue>)  [unwired: 3 in, 2 out]
                  n196 = Bundle By Name(cluster=cluster{"Status":string, "variant":variant} {"Status"="AGGIORNA COMANDI ALIMENTATORE", "variant"=variant}, "variant"=w525) -> (w526:cluster{"Status":string, "variant":variant})
                  n197 = Bundle By Name(cluster=cluster{"Status":string, "variant":variant} {"Status"="AGGIORNA COMANDI ALIMENTATORE", "variant"=variant}, "variant"=w519) -> (w524:cluster{"Status":string, "variant":variant})
                  n198 = Enqueue Element(queue=w529, element=w526) -> ()  [unwired: 2 in, 3 out]
                  n199 = Enqueue Element(queue=w521, element=w524) -> ()  [unwired: 2 in, 3 out]
                }
                frame True {
                  n200 = Unbundle By Name(w563) -> ("ALIMENTATORE 1.RIF V"=w561:dbl)
                  n201 = Unbundle By Name(w562) -> ("V1"=w560:dbl)
                  n202 = Multiply(x=w561, y=w560) -> (x*y=w559:dbl)
                  n203 = Divide(x=w559, y=100.0) -> (x/y=w557:dbl)
                  n204 = To Variant(anything=w557) -> (Variant=w568:variant)
                  n205 = Bundle By Name(cluster=cluster{"state":string, "data":variant} {"state"="", "data"=variant} ("element"), "state"="Calculate Limits", "data"=w568) -> (w565:cluster{"state":string, "data":variant})
                  n206 = Obtain Queue(name (unnamed)="VARIAC_Q", element data type=cluster{"state":string, "data":variant} {"state"="", "data"=variant} ("element")) -> (queue out=w570:refnum<queue>, error out=w569:errorcluster)  [unwired: 3 in, 1 out]
                  n207 = Enqueue Element(queue=w570, element=w565, error in (no error)=w569) -> ()  [unwired: 1 in, 3 out]
                }
              }
              n208 = Multiply(x=w510, y=w511) -> (x*y=w509:dbl)
              n209 = Unbundle By Name(w492) -> ("Control.Control Type"=w491:T20)
              n210 = Divide(x=w509, y=100.0) -> (x/y=w507:dbl)
              n211 = Bundle By Name(cluster=w492, "Control.Control Type"=w490, "Control.Set"=w507, "PID"=w495, "Control.Inverti senso di rotazione"=w484) -> (w496:T15)
              n212 = Equal?(x=w491, y=w490) -> (x = y?=w487:bool)
              n213 = Not(x=w487) -> (.not. x?=w486:bool)
              n214 = global write "Global CAMBIO CTRL FRENO.vi" "CAMBIO CTRL IN CORSO"(w486) -> ()
              n215 = Obtain Queue(name (unnamed)="FRENI", element data type=T6 {"Message"="", "Message Data"=variant} ("Message Cluster")) -> (queue out=w500:refnum<queue>)  [unwired: 3 in, 2 out]
              n216 = Bundle By Name(cluster=cluster{"Status":string, "variant":variant} {"Status"="AGGIORNA COMANDI FRENO", "variant"=variant}, "variant"=w496) -> (w497:cluster{"Status":string, "variant":variant})
              n217 = Select(t="ATTENDI AGGIORNAMENTO VAR GLOB", s=w479, f="ATTENDI TEMPO STEP" ("t")) -> (s? t:f=w480:string)
              n218 = Select(t=w480, s=w487, f="ATTENDI CAMBIO CONTROLLO") -> (s? t:f=w489:string)
              n219 = Enqueue Element(queue=w500, element=w497) -> ()  [unwired: 2 in, 3 out]
            }
            frame "Wait procedura" {
              n220 = global read "Global Fine procedure.vi" "Fine procedure?"() -> (w584:bool)
              n221 = Wait (ms)(milliseconds to wait=u32 10) -> ()  [unwired: 1 out]
              n222 = Select(t="Set step", s=w584, f=w583) -> (s? t:f=w582:string)
            }
          }
        }
        n223 = local write "StatoEsegui"(w123) -> ()
        n224 = Bundle By Name(cluster=w121, "IN ESECUZIONE"=TRUE, "IN PAUSA"=w118, "FINE"=w118, "Tstep"=w109) -> (w120:T3)
        n225 = Select(t=cluster{"Status":string, "variant":variant} {"Status"="FINE", "variant"=variant}, s=w128, f=cluster{"Status":string, "variant":variant} {"Status"="ESEGUI", "variant"=variant}) -> (s? t:f=w113:cluster{"Status":string, "variant":variant})
        n226 = Select(t=cluster{"Status":string, "variant":variant} {"Status"="START PROFILO", "variant"=variant}, s=w111, f=w113) -> (s? t:f=w112:cluster{"Status":string, "variant":variant})
        n227 = Enqueue Element(queue=w127, element=w112) -> ()  [unwired: 2 in, 3 out]
      }
      frame "Exit" {
        w591 = TRUE
        n228 = property on="EXIT" class="Bool (strict)"("Val(Sgnl)"=w591) -> ()  [unwired: 2 in, 2 out]
      }
      frame "FINE" {
        w601 = FALSE ("IN ESECUZIONE")
        n229 = Flush Queue(queue=w610) -> (queue out=w606:refnum<queue>)  [unwired: 1 in, 2 out]
        n230 = Unbundle By Name(w598) -> ("stop al termine"=w597:bool)
        n231 = Enqueue Element(queue=w606, element=cluster{"Status":string, "variant":variant} {"Status"="IDLE", "variant"=variant}) -> ()  [unwired: 2 in, 3 out]
        n232 = case shown="True" w597 {
          frame False {
          }
          frame True {
            n233 = Bundle By Name(cluster=cluster{"Status":string, "variant":variant} {"Status"="AGGIUNGI PROCEDURA", "variant"=variant}, "variant"=cluster{"PROCEDURE":T12, "Variant":variant} {"PROCEDURE"=enum."STOP AUTOMATICO", "Variant"=variant}) -> (w617:cluster{"Status":string, "variant":variant})
            n234 = Obtain Queue(name (unnamed)="PROCEDURE", element data type=T6 {"Message"="", "Message Data"=variant} ("Message Cluster")) -> (queue out=w614:refnum<queue>)  [unwired: 3 in, 2 out]
            n235 = Enqueue Element At Opposite End(queue=w614, element=w617) -> ()  [unwired: 2 in, 3 out]
          }
        }
        n236 = Bundle By Name(cluster=w604, "IN ESECUZIONE"=w601, "IN PAUSA"=w601, "FINE"=TRUE) -> (w603:T3)
      }
      frame "IDLE" {
        n237 = Bundle("Caratteristiche step"=w626, "Step profilo"=w624) -> (w627:T21)  [unwired: 1 in]
        n238 = Bundle By Name(cluster=T10 {"Array of elements"=[], "Single element"={"String"="CARICA TABELLA PROFILO", "variant"=variant}, "enque at\nopposite end (F)"=FALSE, "no replications (F)"=FALSE} ("Enqueue cluster"), "Single element.variant"=w627) -> (w628:T10)
        n239 = call <userlib>:"SMQ_MANAGER.vi"("Function"=enum16{"INITIALIZE", "ENQUEUE", "STOP ALL"}."ENQUEUE", "Queue name"="MAIN2_Q", "Enqueue cluster"=w628) -> ()  [unwired: 8 in, 1 out]
      }
      frame "PAUSA PROFILO" {
        w637 = FALSE ("IN ESECUZIONE")
        n240 = Flush Queue(queue=w645) -> ()  [unwired: 1 in, 3 out]
        n241 = Bundle By Name(cluster=w640, "IN ESECUZIONE"=w637, "IN PAUSA"=TRUE, "FINE"=w637) -> (w639:T3)
      }
      frame "SETTINGS PROFILO" {
        n242 = Variant To Data(type=T13 {"Step iniziale"=0, "N°cicli"=0, "stop al termine"=FALSE} ("Settings profilo"), Variant=w655) -> (data=w652:T13)  [unwired: 1 in, 1 out]
        "Settings profilo" <- w652
      }
      frame "START PROFILO" {
        # "BENAZZATO: RITARDO INTRODOTTO PER EVITARE UNA RACE CONDITION DELLA MORTE (6 ORE PER TROVARE IL BACO). \nSE, DA PROFILO SI EFFETTUANO DUE MISURE DI RESISTENZA UNA DOPO L'ALTRA, VENIVANO PER ERRORE INSERITE\nIN CODA SU GESTIONE PROCEDURA DUE ELEMENTI \"ESTRAI PROCEDURE\" CHE MI FACEVANO SALTARE L'ESECUZIONE\nDI ALCUNE PROCEDURE.\nLA PRIMA SERIE DI PROCEDURE DOVUTA ALLA PRIMA MISURA DI RESISTENZA TERMINAVA CON \"START PROFILO\" E \"FINE\".\nSTART PROFILO FACEVA PARTIRE L'AGGIUNGI PROCEDURA PRIMA CHE IL COMANDO DI FINE VENISSE ESEGUITO. LA SECONDA\nPROCEDURA MI PARTIVA CON UNO STOP AUTOMATICO CHE DI DEFAULT AGGIUNGE IN CODA UN ESTRAI PROCEDURA. MI RITROVAVO\nPOI, QUANDO TORNAVO SU ESEGUI, AD ESEGUIRE UN FINE CHE MI METTEVA IN CODA ESTRAI PROCEDURA ---> SALTAVO LO \nSTOP AUTOMATICO ---> PARTIVA L'APERTURA DEI TELERUTTORI ---> ARRIVAVA L'ESTRAI PROCEDURA INSERITA QUANDO ERA\nSTATA AGGIUNTA LA PROCEDURA DI STOP AUTOMATICO ---> SALTAVO LA SECONDA MISURA DI RESISTENZA ---> IL SITEMA RIPARTIVA"
        # "riprendi il passo messo in pausa inizializzando il tempo step per riprenderlo da dove era stato interrotto,"
        n243 = Unbundle By Name(w666) -> ("Misura resistenza ?"=w664:bool)
        n244 = Unbundle By Name(w675) -> ("Tstep"=w667:dbl, "IN PAUSA"=w674:bool)
        n245 = Enqueue Element(queue=w679, element=cluster{"Status":string, "variant":variant} {"Status"="ESEGUI", "variant"=variant}) -> ()  [unwired: 2 in, 3 out]
        n246 = Bundle By Name(cluster=w666, "Tempo Step[s]"=w667) -> (w668:T7)
        n247 = Unbundle By Name(w662) -> ("#ripetizione in corso"=w661:i32)
        n248 = case shown="False" w664 {
          tunnel: w673 -> [w689 w692]
          tunnel: [w687 w692] -> w669
          tunnel: w668 -> [w688 _]
          tunnel: w663 -> [w690 _]
          tunnel: w661 -> [w686 _]
          frame False {
            # "reinserisci lo step nel profilo nella posizione corretta per\nessere ripreso"
            n249 = Equal To 0?(x=w686) -> (x = 0?=w684:bool)
            n250 = Unbundle By Name(w690) -> ("Step iniziale"=w691:i32)  [unwired: 1 out]
            n251 = Decrement(x=w691) -> (x-1=w685:i32)
            n252 = Select(t=w685, s=w684, f=0) -> (s? t:f=w682:i32)
            n253 = Insert Into Array(array=w689, index=w682, new element=w688) -> (w687:T7[])
          }
          frame True {
            # "se lo step era una misura di resistenza, tralascialo"
          }
        }
        n254 = local write "StatoEsegui"("ESTRAI" ("StatoEsegui")) -> ()
        n255 = disable-structure shown="Disabled" {
          frame Disabled {
          }
          frame Enabled {
          }
        }
        n256 = case shown="True" "To Select Wait" {
          frame False {
          }
          frame True {
            n257 = Wait (ms)(milliseconds to wait=u32 2000) -> ()  [unwired: 1 out]
          }
        }
        n258 = Select(t=w669, s=w674, f=w665) -> (s? t:f=w672:T7[])
      }
      frame "STOP PROFILO" {
        n259 = Flush Queue(queue=w695) -> (queue out=w696:refnum<queue>)  [unwired: 1 in, 2 out]
        n260 = Enqueue Element(queue=w696, element=cluster{"Status":string, "variant":variant} {"Status"="FINE", "variant"=variant}) -> ()  [unwired: 2 in, 3 out]
        n261 = local write "StatoEsegui"("ESTRAI" ("StatoEsegui")) -> ()
      }
    }
    "Cluster 2" <- w11
  }
  n262 = while {
    tunnel: w2 -> [w708]
    stop <- w707 stop-if-true
    n263 = event shown="[2] \"Pause Button\": Value Change" {
      selector: _ -> [_ _ _ _ _ _ _]
      dyn-events: _ -> [_ _ _ _ _ _ _]
      timeout: _ -> [_ _ _ _ _ _ _]
      tunnel: w708 -> [_ w709 w711 _ w717 w721 w725]
      tunnel: [_ _ _ TRUE _ _ _] -> w707
      event Timeout {
        n264 = event-data() -> ()  [unwired: 1 in, 3 out]
      }
      event "Play Button": Value Change {
        n265 = event-data() -> ()  [unwired: 1 in, 6 out]
        n266 = Enqueue Element(queue=w709, element=cluster{"Status":string, "variant":variant} {"Status"="START PROFILO", "variant"=variant}) -> ()  [unwired: 2 in, 3 out]
      }
      event "Pause Button": Value Change {
        n267 = event-data() -> ()  [unwired: 1 in, 6 out]
        n268 = Enqueue Element(queue=w711, element=cluster{"Status":string, "variant":variant} {"Status"="PAUSA PROFILO", "variant"=variant}) -> ()  [unwired: 2 in, 3 out]
      }
      event "EXIT": Value Change {
        n269 = event-data() -> ()  [unwired: 1 in, 6 out]
      }
      event "AGGIORNA DATI NOMINALI": Value Change {
        n270 = event-data() -> ()  [unwired: 1 in, 6 out]
        n271 = local read "Data"() -> (w714:T5)
        n272 = Bundle By Name(cluster=cluster{"Status":string, "variant":variant} {"Status"="AGGIORNA DATI NOMINALI", "variant"=variant}, "variant"=w714) -> (w715:cluster{"Status":string, "variant":variant})
        n273 = Enqueue Element(queue=w717, element=w715) -> ()  [unwired: 2 in, 3 out]
      }
      event "CARICA PROFILO": Value Change {
        n274 = event-data() -> ()  [unwired: 1 in, 6 out]
        n275 = Bundle By Name(cluster=cluster{"Status":string, "variant":variant} {"Status"="CARICA PROFILO", "variant"=variant}, "variant"="NOME PROFILO") -> (w719:cluster{"Status":string, "variant":variant})
        n276 = Enqueue Element(queue=w721, element=w719) -> ()  [unwired: 2 in, 3 out]
      }
      event "AGGIORNA SETTINGS AVVIO": Value Change {
        n277 = event-data() -> ()  [unwired: 1 in, 6 out]
        n278 = local read "Modalità avvio"() -> (w722:T4)
        n279 = Bundle By Name(cluster=cluster{"Status":string, "variant":variant} {"Status"="AGGIORNA SETTINGS AVVIO", "variant"=variant}, "variant"=w722) -> (w723:cluster{"Status":string, "variant":variant})
        n280 = Enqueue Element(queue=w725, element=w723) -> ()  [unwired: 2 in, 3 out]
      }
    }
  }
